vi "Filtra curva experimental.vi"(8 "error in (no error)":errorcluster, 11 "Y":dbl[](array[numeric])) -> (0 "error out":errorcluster, 1 "Tamaño de Y filtrada":i32, 3 "Y Filtrada":dbl[](array[numeric]))   [LabVIEW 2025, in "Control de MaP.lvlib"]
uses:
  Control de MaP.lvlib
  <vilib>/Analysis/3filter.llb/Filter Passband Type.ctl
  <vilib>/Analysis/3filter.llb/Butterworth Filter (DBL).vi
  <vilib>/Analysis/NI_AALBase.lvlib
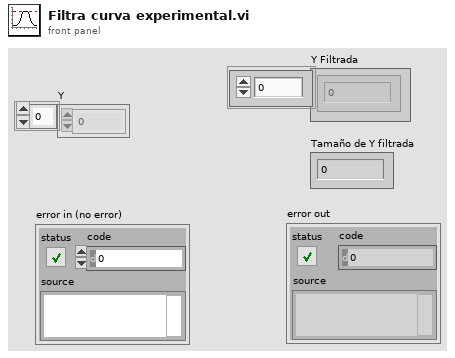
[diagram p1: front panel]
types:
  T1 = typedef "NI_AALBase.lvlib/Filter Passband Type.ctl" = enum32{"Lowpass", "Highpass", "Bandpass", "Bandstop"}
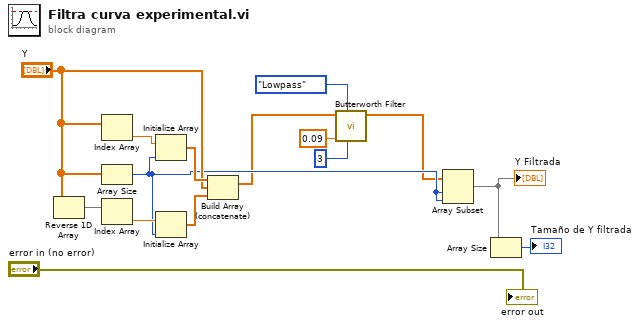
[diagram p0: block diagram]
diagram:
  n1 = Reverse 1D Array(array="Y") -> (reversed array=w13:dbl[])
  n2 = Index Array(array="Y") -> (element=w11:dbl)  [unwired: 1 in]
  n3 = Array Size(array="Y") -> (size(s)=w9:i32)
  n4 = Index Array(array=w13) -> (element=w14:dbl)  [unwired: 1 in]
  n5 = Initialize Array(w11, w9) -> (w12:dbl[])
  n6 = Initialize Array(w14, w9) -> (w15:dbl[])
  n7 = Build Array (concatenate)(w12, "Y", w15) -> (w6:dbl[])
  n8 = call-poly <vilib>:"Butterworth Filter.vi"("order"=3, "filter type"=Filter_Passband_Type."Lowpass", "low cutoff freq: fl"=0.09, "X"=w6) -> ("Filtered X"=w1:dbl[])  [unwired: 4 in, 1 out]
  n9 = Array Subset(array=w1, index=w9, length=w9) -> (w8:dbl[])
  "Y Filtrada" <- w8
  n10 = Array Size(array=w8) -> (size(s)=→"Tamaño de Y filtrada":i32)
  "error out" <- "error in (no error)"
